vi "Yscaling_2_0.vi"(8 "Nano Z Read":dbl, 9 "Current Maxed?":bool, 10 "Y":dbl, 11 "Plane Height":dbl) -> (3 "y scaled":dbl, 4 "Testoutput":dbl)   [LabVIEW 2017]
uses:
  <userlib>/HapticSTM/Feedbackless - Testdata/Project/HapticSTM.lvlib
panel:
  out "force":T1(graph)
  out "Zpos":T2(graph)
  out "appended array":dbl[](array[numeric])
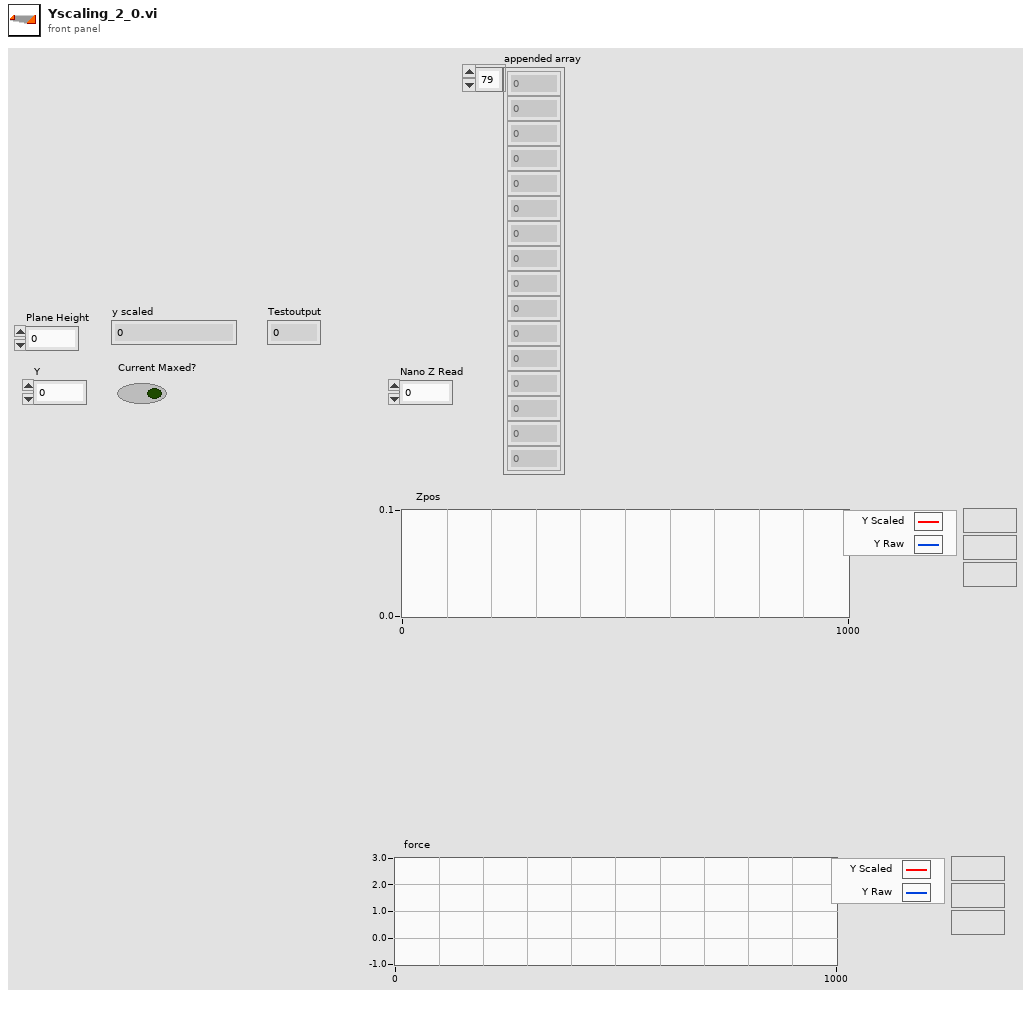
[diagram p1: front panel]
types:
  T1 = cluster{"function return":dbl, "function return":dbl, "function return":dbl}
  T2 = cluster{dbl, "function return":dbl, "function return":dbl}
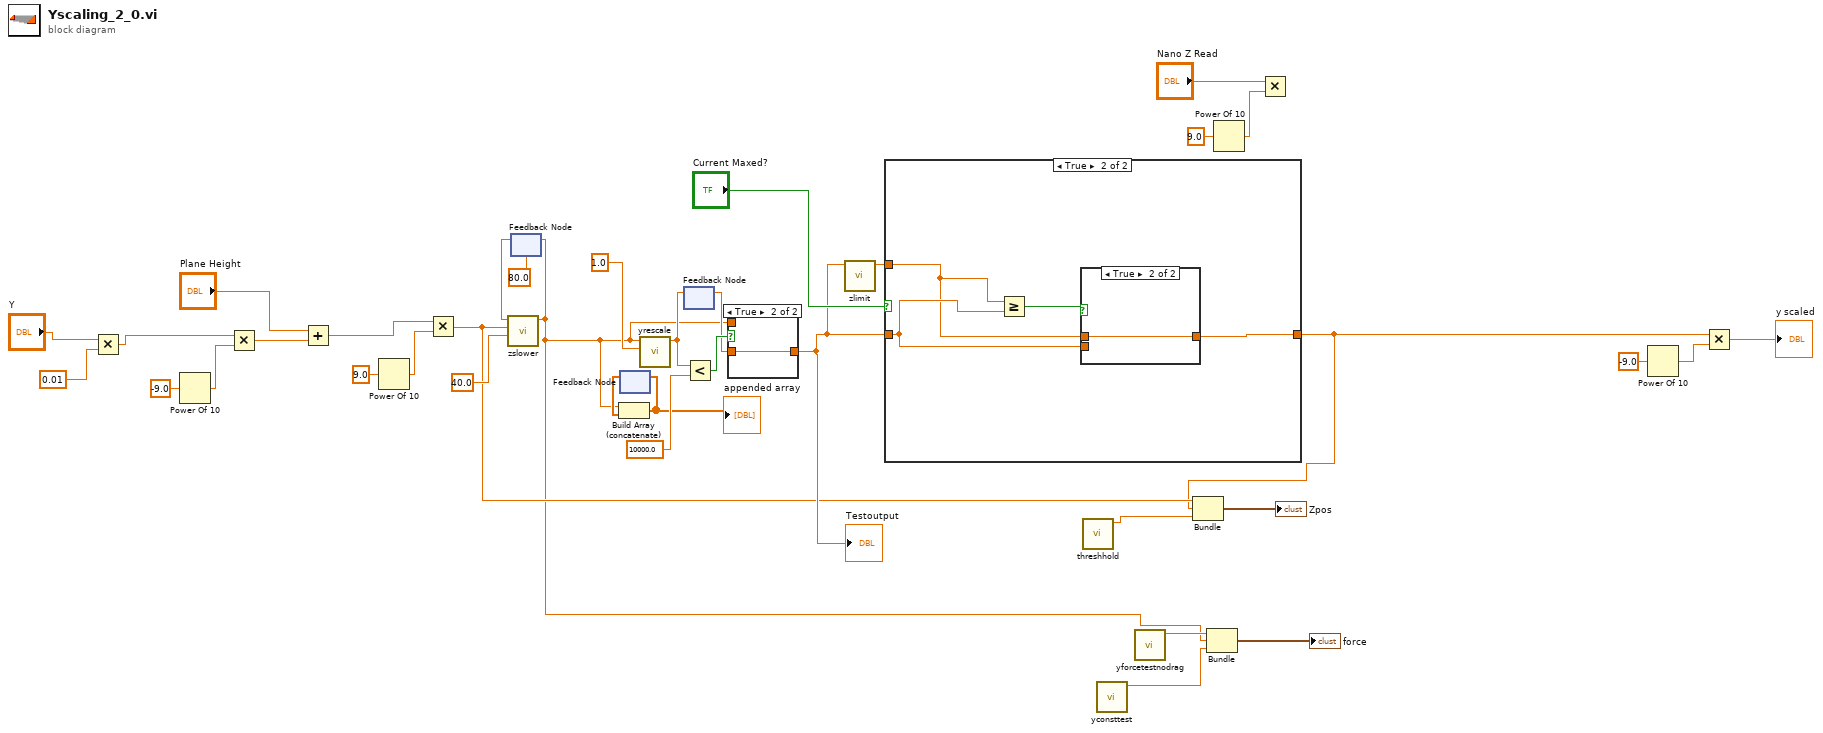
[diagram p0: block diagram]
diagram:
  n1 = Multiply(x="Y", y=0.01) -> (x*y=w33:dbl)
  n2 = Power Of 10(x=-9.0) -> (10^x=w32:dbl)
  n3 = Multiply(x=w33, y=w32) -> (x*y=w34:dbl)
  n4 = Add(x="Plane Height", y=w34) -> (x+y=w37:dbl)
  n5 = Power Of 10(x=9.0) -> (10^x=w36:dbl)
  n6 = Multiply(x=w37, y=w36) -> (x*y=w9:dbl)
  n7 = feedback #1(80.0 ("function return")) -> (w11:dbl)
  n8 = call <userlib>:"zslower.vi"("maxvel"=40.0, "labview_zpos_write"=w9, "nanonis_zpos_read"=w11) -> ("function return"=w2:dbl)  [unwired: 8 in]
  n9 = feedback-in #1(w2) -> ()
  n10 = feedback #2() -> (w13:dbl[])  [unwired: 1 in]
  n11 = Build Array (concatenate)(w2, w13) -> (w14:dbl[])
  "appended array" <- w14
  n12 = feedback-in #2(w14) -> ()
  n13 = call <userlib>:"yrescale.vi"("scalingfactor"=1.0, "ylabview"=w2) -> ("function return"=w3:dbl)  [unwired: 9 in]
  n14 = feedback-in #3(w3) -> ()
  n15 = feedback #3() -> (w18:dbl)  [unwired: 1 in]
  n16 = Less?(x=w3, y=10000.0) -> (x < y?=w19:bool)
  n17 = case shown="True" w19 {
    tunnel: [w38 w39] -> w21
    tunnel: w18 -> [_ w39]
    tunnel: w2 -> [w38 _]
    frame False {
    }
    frame True {
    }
  }
  "Testoutput" <- w21
  n18 = call <userlib>:"zlimit.vi"("yscaledinput"=w21) -> ("function return"=w22:dbl)  [unwired: 10 in]
  n19 = case shown="True" "Current Maxed?" {
    tunnel: [w40 w44] -> w8
    tunnel: w21 -> [w40 w42]
    tunnel: w22 -> [_ w41]
    frame False {
    }
    frame True {
      n20 = Greater Or Equal?(x=w41, y=w42) -> (x >= y?=w43:bool)
      n21 = case shown="True" w43 {
        tunnel: w41 -> [_ w46]
        tunnel: [w45 w46] -> w44
        tunnel: w42 -> [w45 _]
        frame False {
        }
        frame True {
        }
      }
    }
  }
  n22 = call <userlib>:"threshhold.vi"() -> ("function return"=w6:dbl)  [unwired: 11 in]
  n23 = call <userlib>:"yconsttest.vi"() -> ("function return"=w1:dbl)  [unwired: 11 in]
  n24 = call <userlib>:"yforcetestnodrag.vi"() -> ("function return"=w4:dbl)  [unwired: 11 in]
  n25 = Bundle(w9, "function return"=w8, "function return"=w6) -> (→"Zpos":T2)  [unwired: 1 in]
  n26 = Bundle("function return"=w4, "function return"=w2, "function return"=w1) -> (→"force":T1)  [unwired: 1 in]
  n27 = Power Of 10(x=9.0) -> (10^x=w17:dbl)
  n28 = Multiply(x="Nano Z Read", y=w17) -> ()  [unwired: 1 out]
  n29 = Power Of 10(x=-9.0) -> (10^x=w25:dbl)
  n30 = Multiply(x=w8, y=w25) -> (x*y=→"y scaled":dbl)
